vi "Render.vi"(7 "Renderer":refnum<class "Renderer.lvclass">, 8 "error in (no error)":errorcluster, 10 "Camera":refnum<class "Camera.lvclass">, 11 "Planet in":refnum<class "Planet.lvclass">) -> (0 "error out":errorcluster)   [LabVIEW 2021, in "Planet.lvclass"]
uses:
  Planet.lvclass
  C:/dev/LabVIEW/LabMelee/Source/Application Specific/Element/Element.lvclass
  Camera/Camera.lvclass
  Renderer/Renderer.lvclass
  Element/Element.lvclass/Element.ctl
  Motion/Motion.lvclass/Motion.ctl
  Planet.lvclass/Planet.ctl
  Camera/Camera.lvclass/Camera.ctl
  Re-use Libraries/Vector 2D/Vector 2D.lvclass/Vector 2D.ctl
  Renderer/Renderer.lvclass/Renderer.ctl
  Texture/Texture.lvclass/Texture.ctl
  Re-use Libraries/Vector 2D/Vector 2D.lvclass
  Resource Manager/Resource Manager.lvclass
  Element/Element.lvclass
  LabSDL2/Source/Libraries/LibSDL2 Wrapper/LibSDL2.lvlib
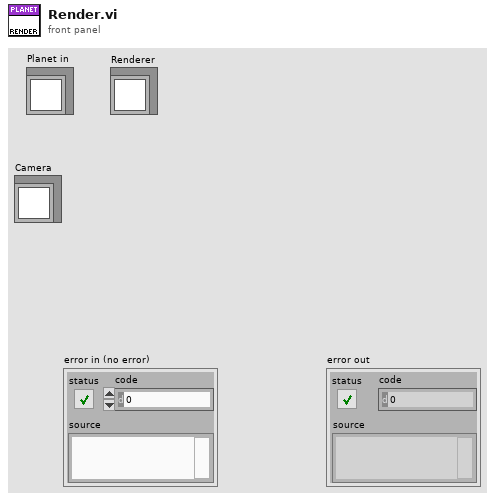
[diagram p1: front panel]
types:
  T1 = typedef "LibSDL2.lvlib/Rectangle.ctl" = cluster{"x":i32, "y":i32, "Width":i32, "Height":i32}
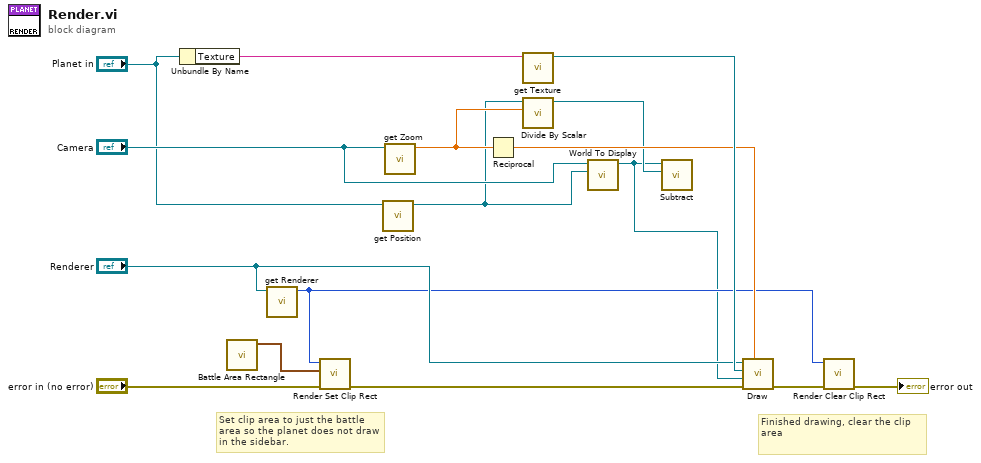
[diagram p0: block diagram]
diagram:
  # "Finished drawing, clear the clip area"
  # "Set clip area to just the battle area so the planet does not draw in the sidebar."
  n1 = Unbundle By Name("Planet in") -> ("Texture"=w16:string)
  n2 = call "Battle Area Rectangle.vi"() -> ("Viewport"=w3:T1)  [unwired: 11 in]
  n3 = call-dynamic "get Renderer.vi"("Renderer in"="Renderer") -> ("Renderer"=w4:u32)  [unwired: 10 in]
  n4 = call "Render Set Clip Rect.vi"("error in"="error in (no error)", "Rectangle"=w3, "Renderer Pointer"=w4) -> ("error out"=w7:errorcluster)  [unwired: 7 in, 1 out]
  n5 = call "get Position.vi"("Element in"="Planet in") -> ("Position"=w1:refnum<class "Vector 2D.lvclass">)  [unwired: 10 in]
  n6 = call "get Zoom.vi"("Camera in"="Camera") -> ("Zoom Level"=w12:sgl)  [unwired: 10 in]
  n7 = Reciprocal(x=w12) -> (1/x=w14:sgl)
  n8 = call "get Texture.vi"("Texture Name"=w16) -> ("Texture"=w15:refnum<class "Texture.lvclass">)  [unwired: 10 in]
  n9 = call "Divide By Scalar.vi"("x"=w12, "A"=w1) -> ("Ax"=w11:refnum<class "Vector 2D.lvclass">)  [unwired: 9 in]
  n10 = call "World To Display.vi"("World Position"=w1, "Camera in"="Camera") -> ("Display Position"=w2:refnum<class "Vector 2D.lvclass">)  [unwired: 9 in]
  n11 = call "Subtract.vi"("B"=w11, "A"=w2) -> ()  [unwired: 9 in, 1 out]
  n12 = call "Draw.vi"("Scale"=w14, "error in (no error)"=w7, "Destination"=w2, "Texture"=w15, "Renderer"="Renderer") -> ("error out"=w6:errorcluster)  [unwired: 6 in]
  n13 = call "Render Clear Clip Rect.vi"("error in"=w6, "Renderer Pointer"=w4) -> ("error out"=→"error out":errorcluster)  [unwired: 8 in, 1 out]
